vi "ConfigureDataRecorder.vi"(0 "System no.":i32=1, 1 "Axes":string[](array[string]), 2 "Analog Input":i32=1, 3 "Record Option for Optical Channel":i32=150, 4 "Record Table rate":i32=20, 5 "error in (no error)":errorcluster) -> (14 "Rec. table IDs Out":i32[](array[numeric]), 19 "error out":errorcluster)   [LabVIEW 2014]
doc: "This VI configures the data recorder to record the positions of the scan axis and the step axis as well as the value of the analog input."
panel:
  # "Configure the data recorder to record axes positions\nand value of analog input."
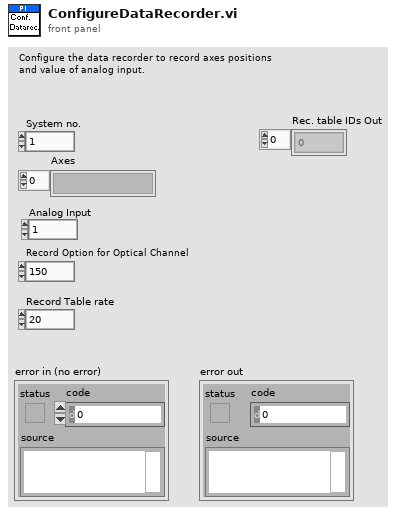
[diagram p1: front panel]
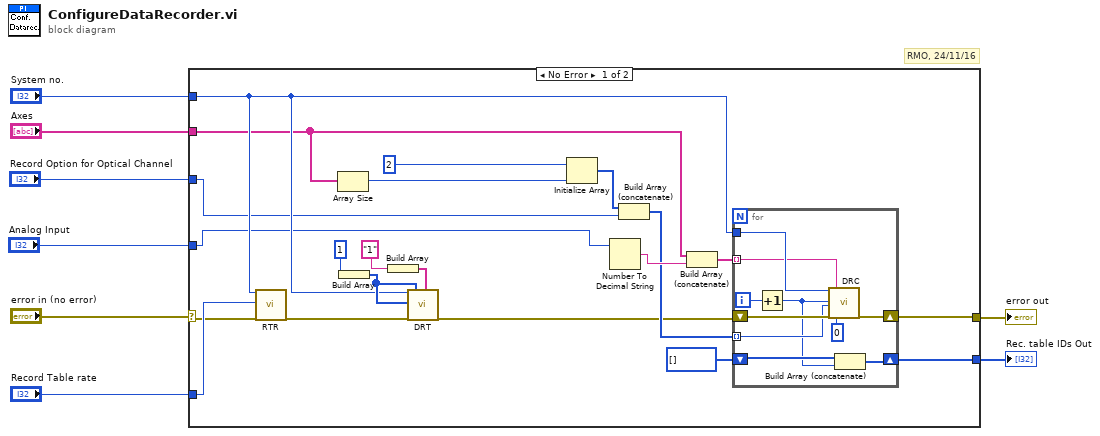
[diagram p0: block diagram]
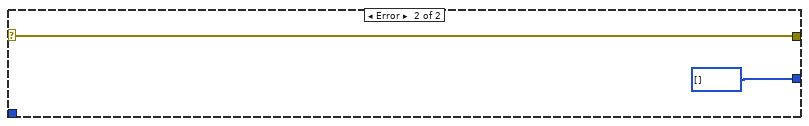
[diagram p2: hidden frame]
diagram:
  # "RMO, 24/11/16"
  n1 = case shown="No Error" "error in (no error)" {
    selector: "error in (no error)" -> [w12 w41]
    tunnel: [w9 w41] -> w8
    tunnel: [w18 i32[] []] -> w6
    tunnel: "System no." -> [w17 _]
    tunnel: "Axes" -> [w16 _]
    tunnel: "Analog Input" -> [w15 _]
    tunnel: "Record Option for Optical Channel" -> [w14 _]
    tunnel: "Record Table rate" -> [w13 _]
    frame No Error {
      n2 = call "RTR.vi"("System no."=w17, "Table rate"=w13, "error in"=w12) -> ("error out"=w11:errorcluster)  [unwired: 16 out]
      n3 = Array Size(array=w16) -> (size(s)=w24:i32)
      n4 = Build Array(1) -> (w28:i32[])
      n5 = Build Array("1") -> (w26:string[])
      n6 = call "DRT.vi"("System no."=w17, "DataRecorderTable"=w28, "error in"=w11, "Trigger source"=w28, "Value"=w26) -> ("error out"=w10:errorcluster)  [unwired: 14 out]
      n7 = Initialize Array(2, w24) -> (w23:i32[])
      n8 = Number To Decimal String(number=w15) -> (decimal integer string=w22:string)  [unwired: 1 out]
      n9 = Build Array (concatenate)(w23, w14) -> (w20:i32[])
      n10 = Build Array (concatenate)(w16, w22) -> (w21:string[])
      n11 = for {
        shift-right: [w38] -> w9
        shift-left: w10 -> [w39]
        tunnel: w17 -> [w37]
        tunnel: w20 -> [w35] mode=indexing
        tunnel: w21 -> [w33] mode=indexing
        shift-right: [w30] -> w18
        shift-left: i32[] [] -> [w32]
        i -> [w36]
        n12 = Increment(x=w36) -> (x+1=w31:i32)
        n13 = call "DRC.vi"("System no."=w37, "Rec. table"=w31, "Rec. option"=w35, "error in"=w39, "Source ID"=w33, "Trigger option"=0) -> ("error out"=w38:errorcluster)  [unwired: 13 out]
        n14 = Build Array (concatenate)(w32, w31) -> (w30:i32[])
      }
    }
    frame Error {
    }
  }
  "error out" <- w8
  "Rec. table IDs Out" <- w6
